vi "Read_Write_Local_table.vi"(3 "Mode":T8, 4 "Ch Values in":T1[](array[typedef]) {"New Value" format="%.2f"}, 5 "Channels Descriptions In":T2[](array[typedef]) {"Duty" format="%016b"; "D" format="%#_5g"; "C" format="%#_5g"; "B" format="%#_5g"; "A" format="%#_5g"}) -> (0 "Ch Names":string[](array[string]), 1 "Ch Values Out":T1[](array[typedef]) {"New Value" format="%.2f"}, 2 "Channels Descriptions Out":T2[](array[typedef]) {"Duty" format="%016b"; "D" format="%#_5g"; "C" format="%#_5g"; "B" format="%#_5g"; "A" format="%#_5g"})   [LabVIEW 2022 SP3]
uses:
  Anemometry/Anemometry Sub Vis/Controls/Global_mode.ctl
  ADAM Controls/Ch_description_ADAM.ctl
  ADAM Controls/Module_type_ADAM.ctl
  ADAM Controls/Function_ADAM.ctl
  ADAM Controls/Channel_State.ctl
  ADAM Controls/Calib_type_ADAM.ctl
  ADAM Controls/Address.ctl
  ADAM Controls/Update_scan_value.ctl
  <vilib>/Utility/error.llb/Trim Whitespace One-Sided.vi
  Anemometry/Anemometry Sub Vis/Globals/Constants_global.vi
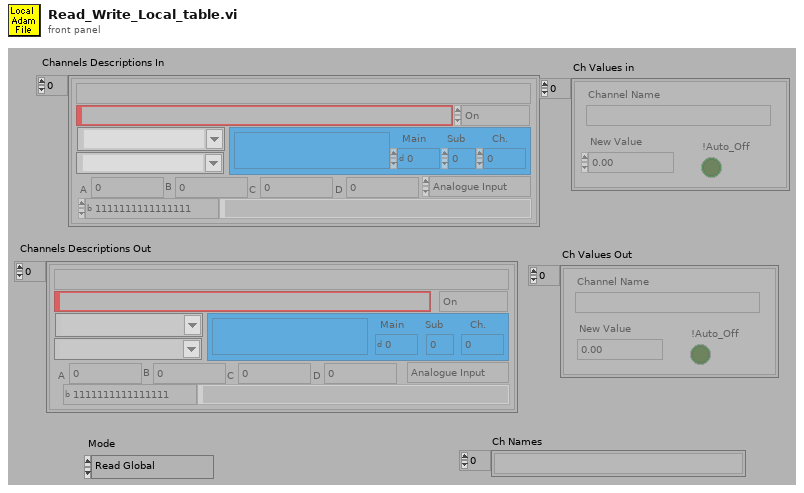
[diagram p1: front panel]
types:
  T1 = typedef "Update_scan_value.ctl" = cluster{"Channel Name":string, "New Value":dbl, "!Auto_Off":bool}
  T2 = typedef "Ch_description_ADAM.ctl" = cluster{"Ch Name":string, "Type":T3, "Function":T4, "Ch State":T5, "Calibration type":T6, "A":dbl, "B":dbl, "C":dbl, "D":dbl, "Comments":string, "Address":T7, "String":string, "Duty":u16}
  T3 = typedef "Module_type_ADAM.ctl" = string
  T4 = typedef "Function_ADAM.ctl" = enum16{"Analogue Input", "Digital Input", "Event counter", "Event rate", "Analogue Output", "Digital Output", "Relay Output"}
  T5 = typedef "Channel_State.ctl" = enum16{"On", "Off", "Always On", "Always Off"}
  T6 = typedef "Calib_type_ADAM.ctl" = string
  T7 = typedef "Address.ctl" = cluster{"Main":i32, "Ch.":i32, "Sub":i32, "Port Name":string}
  T8 = typedef "Global_mode.ctl" = enum16{"Read Global", "Load Global From File", "Write Global to File"}
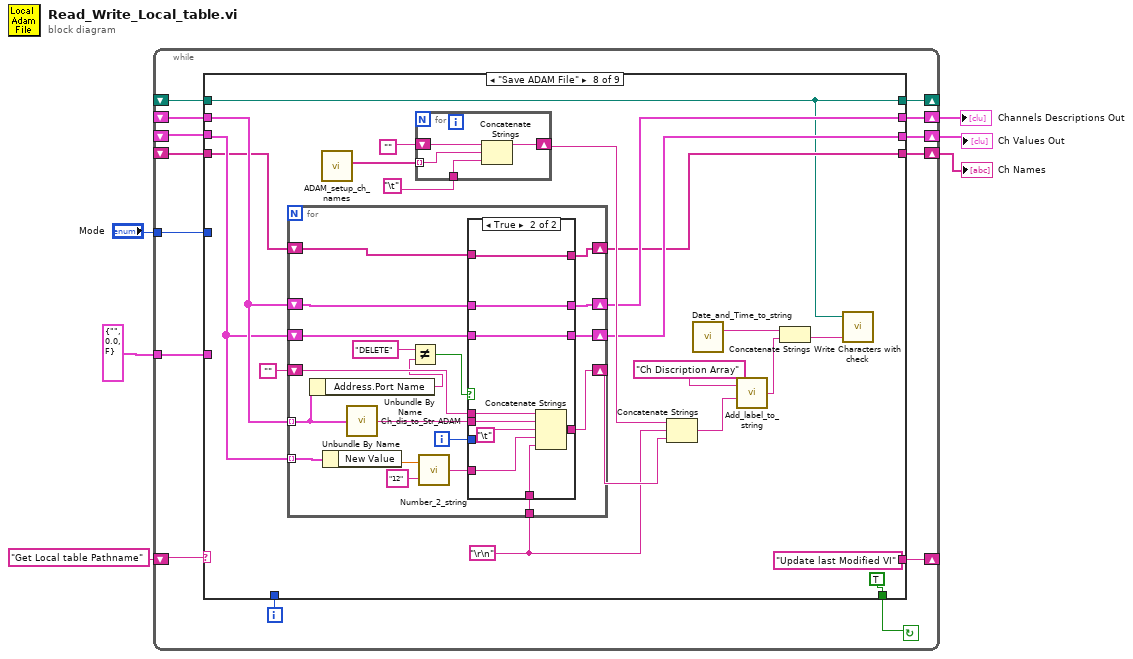
[diagram p0: block diagram]
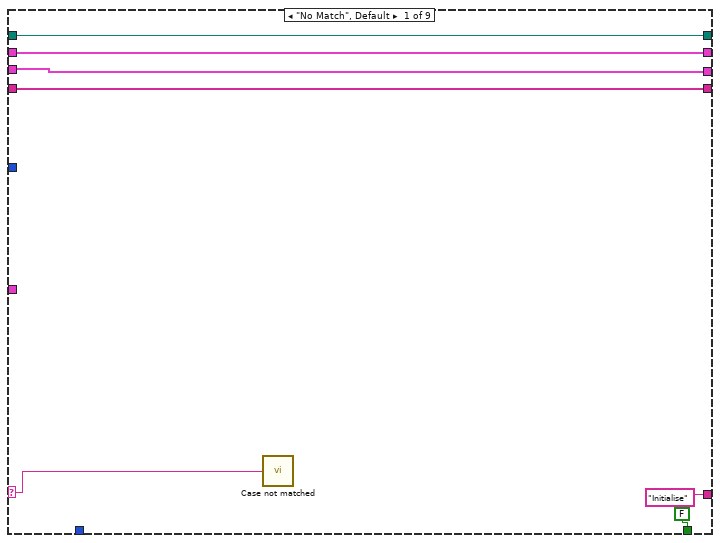
[diagram p2: hidden frame]
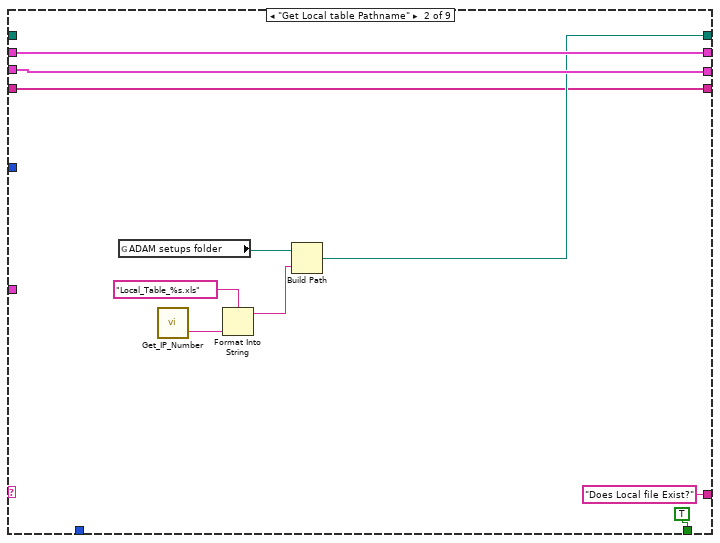
[diagram p3: hidden frame]
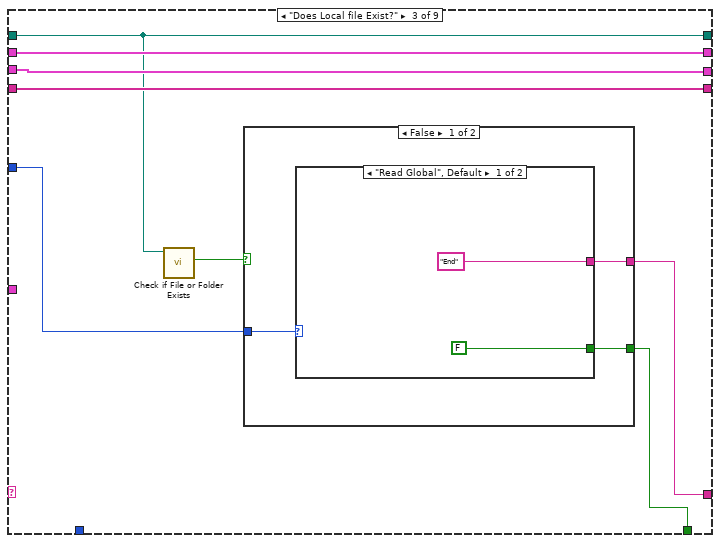
[diagram p4: hidden frame]
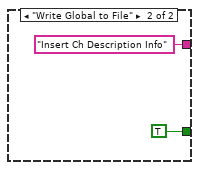
[diagram p5: hidden frame]
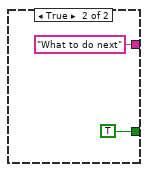
[diagram p6: hidden frame]
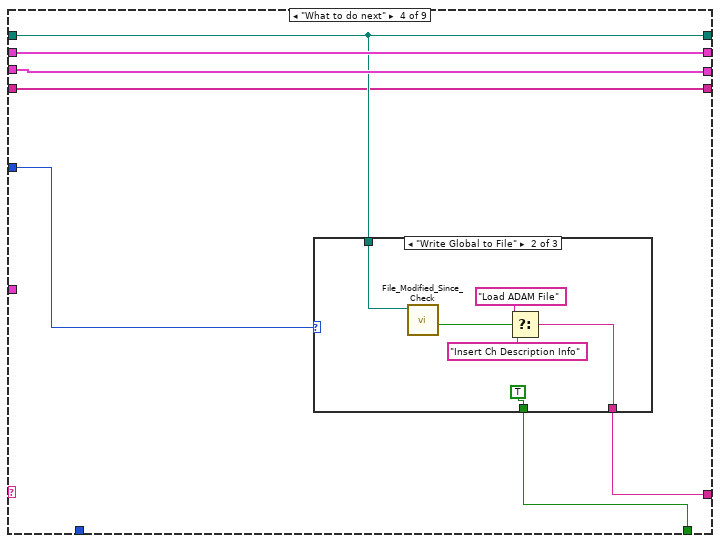
[diagram p7: hidden frame]
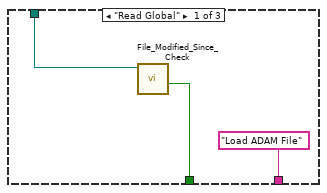
[diagram p8: hidden frame]
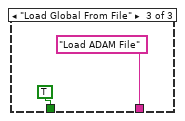
[diagram p9: hidden frame]
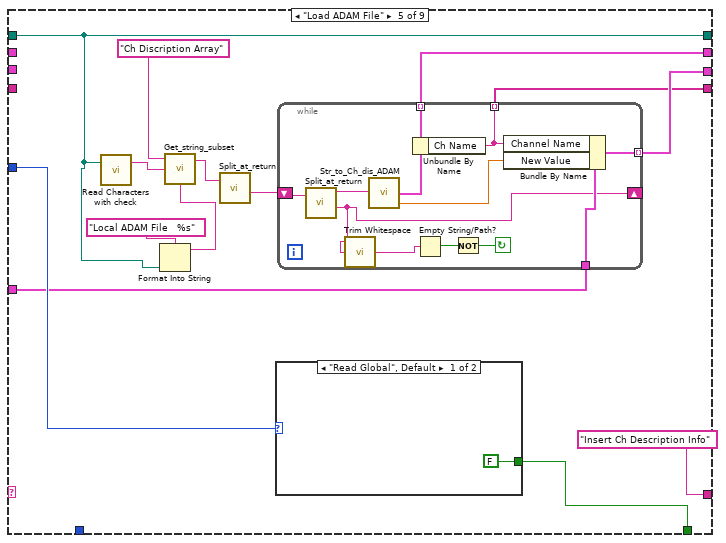
[diagram p10: hidden frame]
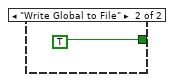
[diagram p11: hidden frame]
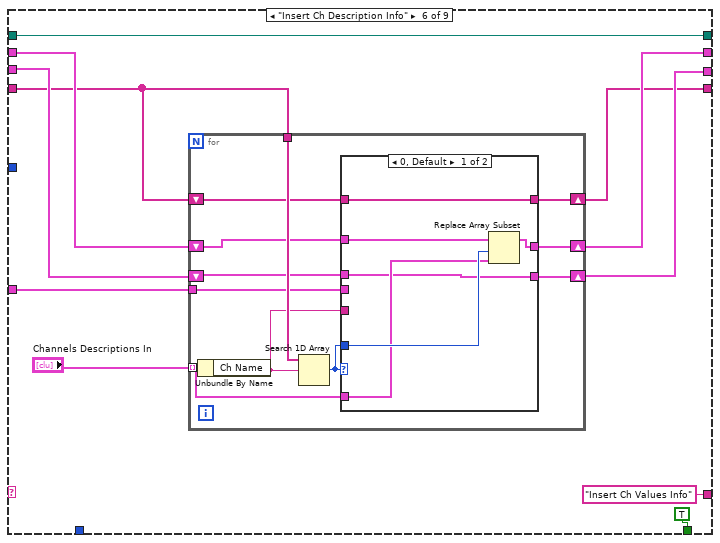
[diagram p12: hidden frame]
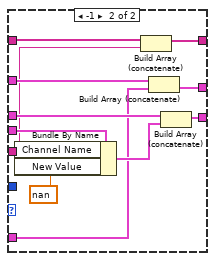
[diagram p13: hidden frame]
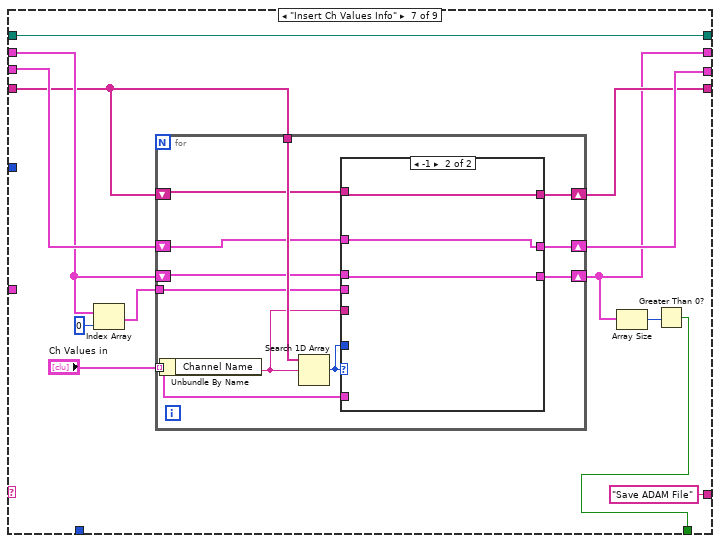
[diagram p14: hidden frame]
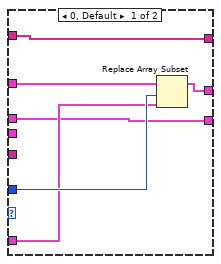
[diagram p15: hidden frame]
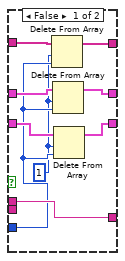
[diagram p16: hidden frame]
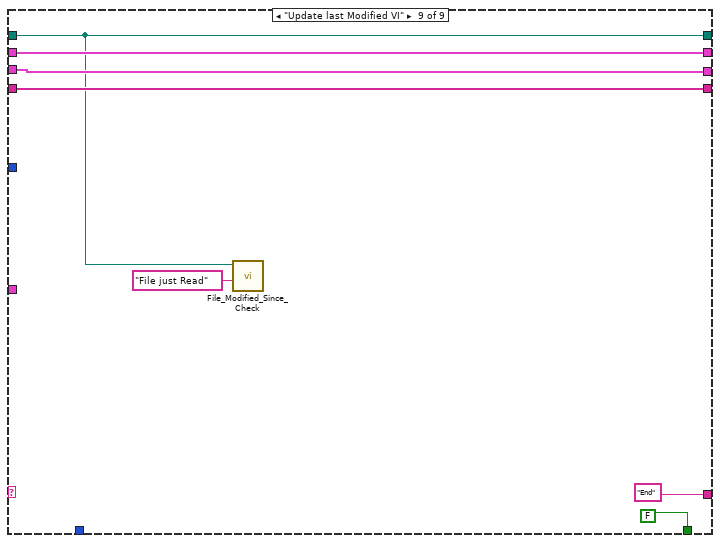
[diagram p17: hidden frame]
diagram:
  n1 = while {
    shift-left: _ -> [w7]
    shift-right: [w8] -> w1
    tunnel: T1 {"Channel Name"="", "New Value"=0.0, "!Auto_Off"=FALSE} ("Update Scan Value Cluster") -> [w9]
    shift-left: _ -> [w11]
    shift-right: [w12] -> w2
    shift-left: _ -> [w13]
    shift-right: [w14] -> w4
    shift-left: _ -> [w17]
    shift-right: [w16] -> _
    tunnel: "Mode" -> [w18]
    shift-left: "Get Local table Pathname" -> [w15]
    shift-right: [w19] -> _
    i -> [w10]
    stop <- w20 continue-if-true
    n2 = case shown="\"Save ADAM File\"" w15 {
      selector: w15 -> [w21 _ _ _ _ _ _ _ _]
      tunnel: [FALSE TRUE w41 w58 w80 TRUE ("Modified?") w139 TRUE FALSE] -> w20
      tunnel: ["Initialise" "Does Local file Exist?" w42 w55 "Insert Ch Description Info" "Insert Ch Values Info" "Save ADAM File" "Update last Modified VI" "End"] -> w19
      tunnel: w18 -> [_ _ w43 w59 w81 _ _ _ _]
      tunnel: w17 -> [w26 _ w39 w57 w74 w102 w150 w172 w235]
      tunnel: [w26 w33 w39 w57 w74 w102 w150 w172 w235] -> w16
      tunnel: [w27 w36 w45 w61 w82 w107 w141 w177 w239] -> w14
      tunnel: w13 -> [w27 w36 w45 w61 _ w109 w146 w180 w239]
      tunnel: [w23 w35 w44 w60 w78 w106 w145 w178 w237] -> w12
      tunnel: w11 -> [w23 w35 w44 w60 _ w108 w147 w179 w237]
      tunnel: w10 -> [_ _ _ _ _ _ _ _ _]
      tunnel: w9 -> [_ _ _ _ w79 w105 _ _ _]
      tunnel: [w22 w31 w40 w56 w77 w100 w142 w175 w236] -> w8
      tunnel: w7 -> [w22 w31 w40 w56 _ w101 w143 w176 w236]
      frame "No Match", Default {
        n3 = call "Case not matched.vi"("Case Name not Matched"=w21) -> ()
      }
      frame "Get Local table Pathname" {
        n4 = global read "Constants_global.vi" "ADAM setups folder"() -> (w34:path)
        n5 = call "Get_IP_Number.vi"() -> ("bestAvailableName"=w29:string)  [unwired: 1 out]
        n6 = Format Into String(format string="Local_Table_%s.xls" ("name or relative path"), w29) -> (resulting string=w28:string)  [unwired: 2 in, 1 out]
        n7 = Build Path(base path=w34, name or relative path=w28) -> (appended path=w33:path)
      }
      frame "Does Local file Exist?" {
        n8 = call <vilib>:"Check if File or Folder Exists.vi"("path"=w39) -> ("file or folder exists?"=w38:bool)  [unwired: 1 in, 9 out]
        n9 = case shown="False" w38 {
          tunnel: w43 -> [w48 _]
          tunnel: [w47 "What to do next"] -> w42
          tunnel: [w46 TRUE] -> w41
          frame False {
            n10 = case shown="\"Read Global\", Default" w48 {
              tunnel: ["End" "Insert Ch Description Info"] -> w47
              tunnel: [FALSE TRUE] -> w46
              frame "Read Global", Default {
              }
              frame "Write Global to File" {
              }
            }
          }
          frame True {
          }
        }
      }
      frame "What to do next" {
        n11 = case shown="\"Write Global to File\"" w59 {
          tunnel: w57 -> [w63 w66 _]
          tunnel: [w62 TRUE ("Modified?") TRUE ("Modified?")] -> w58
          tunnel: ["Load ADAM File" w67 "Load ADAM File"] -> w55
          frame "Read Global" {
            n12 = call "File_Modified_Since_Check.vi"("File Path"=w63) -> ("modifiedSinceRead"=w62:bool)  [unwired: 7 in, 1 out]
          }
          frame "Write Global to File" {
            n13 = call "File_Modified_Since_Check.vi"("File Path"=w66) -> ("modifiedSinceRead"=w65:bool)  [unwired: 7 in, 1 out]
            n14 = Select(t="Load ADAM File", s=w65, f="Insert Ch Description Info") -> (s? t:f=w67:string)
          }
          frame "Load Global From File" {
          }
        }
      }
      frame "Load ADAM File" {
        n15 = call "Read Characters with check.vi"("file (use dialog)"=w74) -> ("Read String"=w73:string)  [unwired: 1 in, 1 out]
        n16 = Format Into String(format string="Local ADAM File   %s", w74) -> (resulting string=w75:string)  [unwired: 2 in, 1 out]
        n17 = call "Get_string_subset.vi"("String Name"=w75, "String to split"=w73, "File Label"="Ch Discription Array") -> ("Output string"=w84:string)  [unwired: 1 in, 1 out]
        n18 = call "Split_at_return.vi"("String"=w84) -> ("after substring"=w83:string)  [unwired: 1 in, 3 out]
        n19 = case shown="\"Read Global\", Default" w81 {
          tunnel: [FALSE TRUE] -> w80
          frame "Read Global", Default {
          }
          frame "Write Global to File" {
          }
        }
        n20 = while {
          tunnel: [w89] -> w77 mode=indexing
          tunnel: [w91] -> w78 mode=indexing
          tunnel: w79 -> [w93]
          tunnel: [w94] -> w82 mode=indexing
          shift-left: w83 -> [w97]
          shift-right: [w88] -> _
          stop <- w95 continue-if-true
          n21 = call "Split_at_return.vi"("String"=w97) -> ("before substring"=w96:string, "after substring"=w88:string)  [unwired: 1 in, 2 out]
          n22 = call <vilib>:"Trim Whitespace.vi"("string"=w88) -> ("trimmed string"=w87:string)  [unwired: 1 in]
          n23 = call "Str_to_Ch_dis_ADAM.vi"("String Row"=w96) -> ("Value"=w92:dbl, "Ch Description"=w94:T2)  [unwired: 1 in, 2 out]
          n24 = Unbundle By Name(w94) -> ("Ch Name"=w89:string)
          n25 = Empty String/Path?(string/path=w87) -> (empty?=w90:bool)
          n26 = Not(x=w90) -> (.not. x?=w95:bool)
          n27 = Bundle By Name(cluster=w93, "Channel Name"=w89, "New Value"=w92) -> (w91:T1)
        }
      }
      frame "Insert Ch Description Info" {
        n28 = for {
          tunnel: "Channels Descriptions In" -> [w114] mode=indexing
          tunnel: w101 -> [w121]
          shift-right: [w118] -> w107
          shift-left: w109 -> [w119]
          shift-right: [w117] -> w106
          shift-left: w108 -> [w120]
          tunnel: w105 -> [w116]
          shift-right: [w112] -> w100
          shift-left: w101 -> [w111]
          n29 = Unbundle By Name(w114) -> ("Ch Name"=w115:string)
          n30 = Search 1D Array(1D array=w121, element=w115) -> (index of element=w113:i32)  [unwired: 1 out]
          n31 = case shown="0, Default" w113 {
            tunnel: w120 -> [w123 w135]
            tunnel: w119 -> [w127 w138]
            tunnel: [w126 w137] -> w118
            tunnel: [w123 w136] -> w117
            tunnel: w116 -> [_ w134]
            tunnel: w115 -> [_ w128]
            tunnel: w114 -> [w124 w131]
            tunnel: w113 -> [w125 _]
            tunnel: [w122 w129] -> w112
            tunnel: w111 -> [w122 w130]
            frame 0, Default {
              n32 = Replace Array Subset(array=w127, new element=w124, index=w125) -> (w126:T2[])
            }
            frame -1 {
              n33 = Bundle By Name(cluster=w134, "Channel Name"=w128, "New Value"=nan ("Bundle Element")) -> (w133:T1)
              n34 = Build Array (concatenate)(w130, w128) -> (w129:string[])
              n35 = Build Array (concatenate)(w138, w131) -> (w137:T2[])
              n36 = Build Array (concatenate)(w135, w133) -> (w136:T1[])
            }
          }
        }
      }
      frame "Insert Ch Values Info" {
        n37 = Index Array(array=w146, index=0 ("Index")) -> (element=w144:T2)
        n38 = for {
          tunnel: "Ch Values in" -> [w155] mode=indexing
          tunnel: w143 -> [w162]
          shift-right: [w159] -> w145
          shift-left: w147 -> [w160]
          shift-right: [w158] -> w141
          shift-left: w146 -> [w161]
          tunnel: w144 -> [w157]
          shift-right: [w152] -> w142
          shift-left: w143 -> [w153]
          n39 = Unbundle By Name(w155) -> ("Channel Name"=w156:string)
          n40 = Search 1D Array(1D array=w162, element=w156) -> (index of element=w154:i32)  [unwired: 1 out]
          n41 = case shown="-1" w154 {
            tunnel: w161 -> [w164 w169]
            tunnel: w160 -> [w168 w170]
            tunnel: [w167 w170] -> w159
            tunnel: [w164 w169] -> w158
            tunnel: w157 -> [_ _]
            tunnel: w156 -> [_ _]
            tunnel: w155 -> [w165 _]
            tunnel: w154 -> [w166 _]
            tunnel: w153 -> [w163 w171]
            tunnel: [w163 w171] -> w152
            frame 0, Default {
              n42 = Replace Array Subset(array=w168, new element=w165, index=w166) -> (w167:T1[])
            }
            frame -1 {
            }
          }
        }
        n43 = Array Size(array=w141) -> (size(s)=w140:i32)
        n44 = Greater Than 0?(x=w140) -> (x > 0?=w139:bool)
      }
      frame "Save ADAM File" {
        w174 = "\r\n"
        n45 = for {
          tunnel: w180 -> [w208] mode=indexing
          shift-right: [w212] -> w182
          shift-left: "" -> [w213]
          tunnel: w179 -> [w211] mode=indexing
          shift-right: [w201] -> w178
          shift-left: w179 -> [w202]
          shift-right: [w203] -> w177
          shift-left: w180 -> [w204]
          shift-right: [w198] -> w175
          shift-left: w176 -> [w199]
          tunnel: w174 -> [w197]
          i -> [w200]
          n46 = Unbundle By Name(w208) -> ("Address.Port Name"=w207:string)
          n47 = Unbundle By Name(w211) -> ("New Value"=w210:dbl)
          n48 = call "Ch_dis_to_Str_ADAM.vi"("Ch Description"=w208) -> ("String Row"=w215:string)  [unwired: 4 out]
          n49 = Not Equal?(x="DELETE", y=w207) -> (x != y?=w205:bool)
          n50 = call "Number_2_string.vi"("precision"="12", "number"=w210) -> ("String"=w214:string)
          n51 = case shown="True" w205 {
            tunnel: w215 -> [_ w232]
            tunnel: w214 -> [_ w231]
            tunnel: w213 -> [w224 w230]
            tunnel: [w224 w229] -> w212
            tunnel: w204 -> [w223 w228]
            tunnel: [w222 w228] -> w203
            tunnel: w202 -> [w221 w227]
            tunnel: [w220 w227] -> w201
            tunnel: w200 -> [w217 _]
            tunnel: w199 -> [w219 w226]
            tunnel: [w218 w226] -> w198
            tunnel: w197 -> [_ w225]
            frame False {
              w216 = 1 ("length")
              n52 = Delete From Array(array=w219, length=w216, index=w217) -> (array with subset deleted=w218:string[])  [unwired: 1 out]
              n53 = Delete From Array(array=w223, length=w216, index=w217) -> (array with subset deleted=w222:T2[])  [unwired: 1 out]
              n54 = Delete From Array(array=w221, length=w216, index=w217) -> (array with subset deleted=w220:T1[])  [unwired: 1 out]
            }
            frame True {
              n55 = Concatenate Strings(w230, w232, "\t", w231, w225) -> (w229:string)
            }
          }
        }
        n56 = call "ADAM_setup_ch_names.vi"() -> ("Ch Names"=w189:string[])  [unwired: 1 out]
        n57 = for {
          shift-right: [w193] -> w181
          shift-left: "" -> [w196]
          tunnel: "\t" -> [w194]
          tunnel: w189 -> [w195] mode=indexing
          n58 = Concatenate Strings(w196, w195, w194) -> (w193:string)
        }
        n59 = Concatenate Strings(w181, w174, w182) -> (w185:string)
        n60 = call "Date_and_Time_to_string.vi"() -> ("Date and time (spreadsheet)"=w184:string)  [unwired: 4 in, 1 out]
        n61 = call "Add_label_to_string.vi"("String to write"=w185, "File Label"="Ch Discription Array") -> ("Output string"=w183:string)
        n62 = Concatenate Strings(w184, w183) -> (w173:string)
        n63 = call "Write Characters with check.vi"("String to Write"=w173, "file (use dialog)"=w172) -> ()  [unwired: 2 in, 1 out]
      }
      frame "Update last Modified VI" {
        n64 = call "File_Modified_Since_Check.vi"("mode"="File just Read", "File Path"=w235) -> ()  [unwired: 6 in, 2 out]
      }
    }
  }
  "Channels Descriptions Out" <- w4
  "Ch Values Out" <- w2
  "Ch Names" <- w1
